vi "ParseNEAMAString.vi"(6 "error in (no error)":errorcluster, 8 "Grennich Offset":dbl=-8.0, 9 "String In (NEAMA GGA)":string="$GPGGA,152703.40,3814.751152,N,12130.720799,W,2,07,1.1,-5.47,M,-23.44,M,3.2,0211\n*5E") -> (0 "error out":errorcluster, 3 "NEMA string capture variables Out":T1)   [LabVIEW 2011]
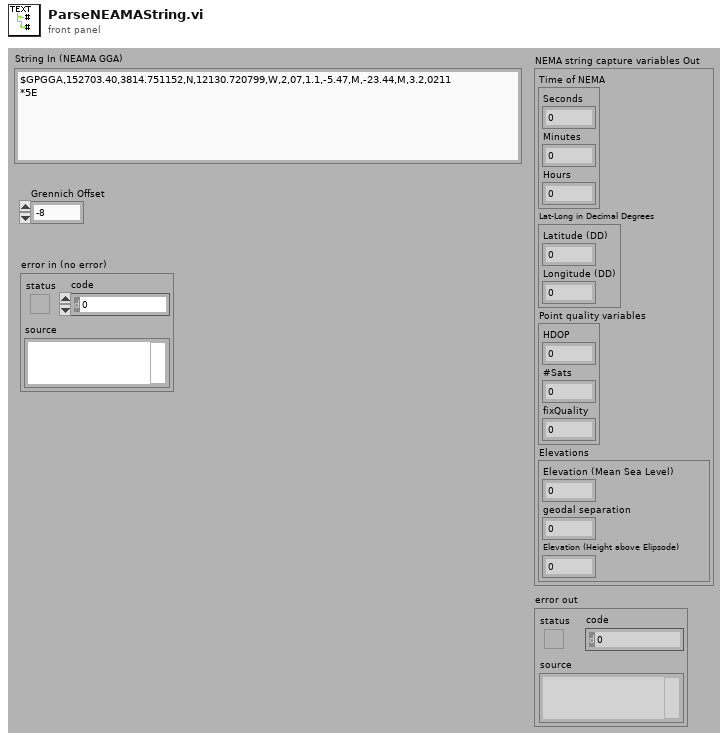
[diagram p1: front panel]
types:
  T1 = cluster{"Time of NEMA":cluster{"Seconds":i32, "Minutes":i32, "Hours":i32}, "Lat-Long in Decimal Degrees":cluster{"Latitude (DD)":dbl, "Longitude (DD)":dbl}, "Point quality variables":cluster{"HDOP":dbl, "#Sats":dbl, "fixQuality":dbl}, "Elevations":cluster{"Elevation (Mean Sea Level)":dbl, "geodal separation":dbl, "Elevation (Height above Elipsode)":dbl}}
  T2 = cluster{"Latitude (DD)":dbl, "Longitude (DD)":dbl}
  T3 = cluster{"Elevation (Mean Sea Level)":dbl, "geodal separation":dbl, "Elevation (Height above Elipsode)":dbl}
  T4 = cluster{"HDOP":dbl, "#Sats":dbl, "fixQuality":dbl}
  T5 = cluster{"Seconds":i32, "Minutes":i32, "Hours":i32}
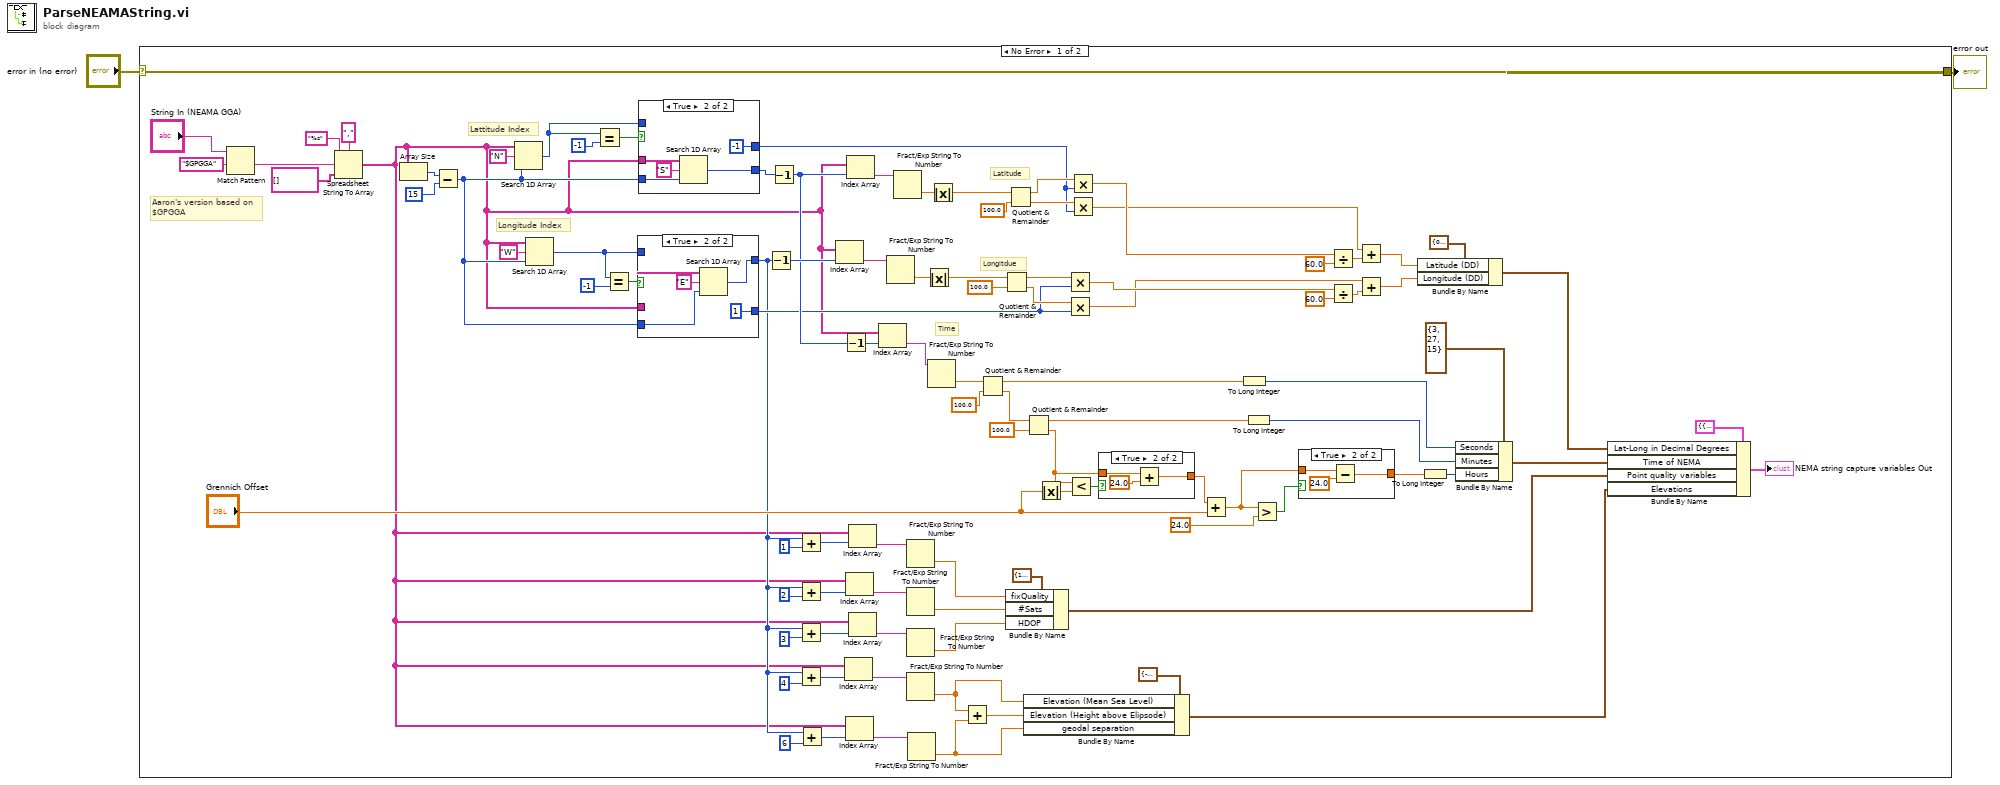
[diagram p0: block diagram]
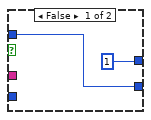
[diagram p3: hidden frame]
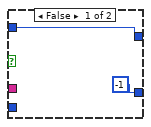
[diagram p4: hidden frame]
diagram:
  n1 = case shown="No Error" "error in (no error)" {
    selector: "error in (no error)" -> [w56 w123]
    tunnel: [w56 w123] -> w1
    frame No Error {
      # "Aaron's version based on\n$GPGGA"
      # "Time"
      # "Longitude Index"
      # "Lattitude Index"
      # "Longitdue"
      # "Latitude"
      n2 = Match Pattern(string="String In (NEAMA GGA)", regular expression="$GPGGA") -> (after substring=w57:string)  [unwired: 4 out]
      n3 = Spreadsheet String To Array(delimiter (Tab)=",", format string="%s", spreadsheet string=w57, array type (2D Dbl)=string[] []) -> (array=w39:string[])
      n4 = Array Size(array=w39) -> (size(s)=w90:i32)
      n5 = Subtract(x=w90, y=15) -> (x-y=w73:i32)
      n6 = Search 1D Array(1D array=w39, element="N", start index (0)=w73) -> (index of element=w72:i32)
      n7 = Search 1D Array(1D array=w39, element="W", start index (0)=w73) -> (index of element=w75:i32)
      n8 = Equal?(x=w72, y=-1) -> (x = y?=w70:bool)
      n9 = Equal?(x=w75, y=-1) -> (x = y?=w77:bool)
      n10 = case shown="True" w77 {
        tunnel: [w113 w114] -> w41
        tunnel: w75 -> [w113 _]
        tunnel: [-1 1] -> w62
        tunnel: w39 -> [_ w116]
        tunnel: w73 -> [_ w115]
        frame False {
        }
        frame True {
          n11 = Search 1D Array(1D array=w116, element="E", start index (0)=w115) -> (index of element=w114:i32)
        }
      }
      n12 = case shown="True" w70 {
        tunnel: [w106 w108] -> w74
        tunnel: w72 -> [w106 _]
        tunnel: [1 -1] -> w63
        tunnel: w73 -> [_ w109]
        tunnel: w39 -> [_ w107]
        frame False {
        }
        frame True {
          n13 = Search 1D Array(1D array=w107, element="S", start index (0)=w109) -> (index of element=w108:i32)
        }
      }
      n14 = Decrement(x=w41) -> (x-1=w94:i32)
      n15 = Decrement(x=w74) -> (x-1=w87:i32)
      n16 = Add(x=w41, y=1 ("index")) -> (x+y=w47:i32)
      n17 = Add(x=w41, y=2 ("index")) -> (x+y=w50:i32)
      n18 = Add(x=w41, y=3 ("index")) -> (x+y=w49:i32)
      n19 = Add(x=w41, y=4 ("index")) -> (x+y=w45:i32)
      n20 = Add(x=w41, y=6 ("index")) -> (x+y=w43:i32)
      n21 = Index Array(array=w39, index=w94) -> (element=w92:string)
      n22 = Decrement(x=w87) -> (x-1=w86:i32)
      n23 = Index Array(array=w39, index=w45) -> (element=w44:string)
      n24 = Index Array(array=w39, index=w43) -> (element=w40:string)
      n25 = Index Array(array=w39, index=w50) -> (element=w54:string)
      n26 = Index Array(array=w39, index=w87) -> (element=w93:string)
      n27 = Index Array(array=w39, index=w47) -> (element=w55:string)
      n28 = Index Array(array=w39, index=w49) -> (element=w53:string)
      n29 = Index Array(array=w39, index=w86) -> (element=w88:string)
      n30 = Fract/Exp String To Number(string=w92) -> (number=w69:dbl)  [unwired: 4 out]
      n31 = Fract/Exp String To Number(string=w93) -> (number=w68:dbl)  [unwired: 4 out]
      n32 = Fract/Exp String To Number(string=w55) -> (number=w26:dbl)  [unwired: 4 out]
      n33 = Fract/Exp String To Number(string=w54) -> (number=w25:dbl)  [unwired: 4 out]
      n34 = Fract/Exp String To Number(string=w53) -> (number=w24:dbl)  [unwired: 4 out]
      n35 = Fract/Exp String To Number(string=w44) -> (number=w22:dbl)  [unwired: 4 out]
      n36 = Fract/Exp String To Number(string=w40) -> (number=w20:dbl)  [unwired: 4 out]
      n37 = Absolute Value(x=w69) -> (abs(x)=w61:dbl)
      n38 = Fract/Exp String To Number(string=w88) -> (number=w85:dbl)  [unwired: 4 out]
      n39 = Absolute Value(x=w68) -> (abs(x)=w60:dbl)
      n40 = Add(x=w22, y=w20) -> (x+y=w21:dbl)
      n41 = Quotient & Remainder(x=w85, y=100.0) -> (x-y*floor(x/y)=w37:dbl, floor(x/y)=w83:dbl)
      n42 = Quotient & Remainder(x=w61, y=100.0) -> (x-y*floor(x/y)=w67:dbl, floor(x/y)=w66:dbl)
      n43 = Bundle By Name(cluster=T4 {"HDOP"=1.1, "#Sats"=7.0, "fixQuality"=2.0} ("Stats of Point quality"), "fixQuality"=w26, "#Sats"=w25, "HDOP"=w24) -> (w13:T4)
      n44 = Quotient & Remainder(x=w60, y=100.0) -> (x-y*floor(x/y)=w65:dbl, floor(x/y)=w64:dbl)
      n45 = Bundle By Name(cluster=T3 {"Elevation (Mean Sea Level)"=-5.47, "geodal separation"=-23.44, "Elevation (Height above Elipsode)"=-28.91} ("Elevations"), "Elevation (Mean Sea Level)"=w22, "Elevation (Height above Elipsode)"=w21, "geodal separation"=w20) -> (w12:T3)
      n46 = Quotient & Remainder(x=w83, y=100.0) -> (x-y*floor(x/y)=w36:dbl, floor(x/y)=w79:dbl)
      n47 = Absolute Value(x="Grennich Offset") -> (abs(x)=w7:dbl)
      n48 = Multiply(x=w67, y=w62) -> (x*y=w29:dbl)
      n49 = Multiply(x=w66, y=w62) -> (x*y=w28:dbl)
      n50 = Less?(x=w79, y=w7) -> (x < y?=w80:bool)
      n51 = Multiply(x=w65, y=w63) -> (x*y=w31:dbl)
      n52 = Multiply(x=w64, y=w63) -> (x*y=w30:dbl)
      n53 = case shown="True" w80 {
        tunnel: [w119 w120] -> w78
        tunnel: w79 -> [w119 w122]
        frame False {
        }
        frame True {
          n54 = Add(x=w122, y=24.0) -> (x+y=w120:dbl)
        }
      }
      n55 = Add(x=w78, y="Grennich Offset") -> (x+y=w4:dbl)
      n56 = To Long Integer(number=w37) -> (32bit integer=w11:i32)
      n57 = To Long Integer(number=w36) -> (32bit integer=w10:i32)
      n58 = Greater?(x=w4, y=24.0) -> (0:w5:bool)
      n59 = case shown="True" w5 {
        tunnel: [w101 w102] -> w3
        tunnel: w4 -> [w101 w104]
        frame False {
        }
        frame True {
          n60 = Subtract(x=w104, y=24.0) -> (x-y=w102:dbl)
        }
      }
      n61 = Divide(x=w31, y=60.0) -> (x/y=w33:dbl)
      n62 = Divide(x=w29, y=60.0) -> (x/y=w34:dbl)
      n63 = Add(x=w30, y=w33) -> (x+y=w18:dbl)
      n64 = Add(x=w28, y=w34) -> (x+y=w17:dbl)
      n65 = Bundle By Name(cluster=T2 {"Latitude (DD)"=0.0, "Longitude (DD)"=0.0} ("Lat-Long in Decimal Degrees"), "Latitude (DD)"=w18, "Longitude (DD)"=w17) -> (w15:T2)
      n66 = To Long Integer(number=w3) -> (32bit integer=w9:i32)
      n67 = Bundle By Name(cluster=T5 {"Seconds"=3, "Minutes"=27, "Hours"=15} ("Time from NEMA"), "Seconds"=w11, "Minutes"=w10, "Hours"=w9) -> (w14:T5)
      n68 = Bundle By Name(cluster=T1 {"Time of NEMA"={"Seconds"=0, "Minutes"=0, "Hours"=0}, "Lat-Long in Decimal Degrees"={"Latitude (DD)"=0.0, "Longitude (DD)"=0.0}, "Point quality variables"={"HDOP"=0.0, "#Sats"=0.0, "fixQuality"=0.0}, "Elevations"={"Elevation (Mean Sea Level)"=0.0, "geodal separation"=0.0, "Elevation (Height above Elipsode)"=0.0}} ("NEMA string capture variables 2"), "Lat-Long in Decimal Degrees"=w15, "Time of NEMA"=w14, "Point quality variables"=w13, "Elevations"=w12) -> (→"NEMA string capture variables Out":T1)
    }
    frame Error {
    }
  }
  "error out" <- w1
